vi "Read PortID.vi"(8 "error in (no error)":errorcluster, 11 "FlexLogger_gRPC in":refnum<class "FlexLogger_gRPC.lvclass">) -> (0 "error out":errorcluster, 2 "PortID":u32, 3 "FlexLogger_gRPC out":refnum<class "FlexLogger_gRPC.lvclass">)   [LabVIEW 2020, in "FlexLogger_gRPC.lvlib" / "FlexLogger_gRPC.lvclass"]
uses:
  FlexLogger_gRPC.lvclass
  FlexLogger_gRPC.lvclass/FlexLogger_gRPC.ctl
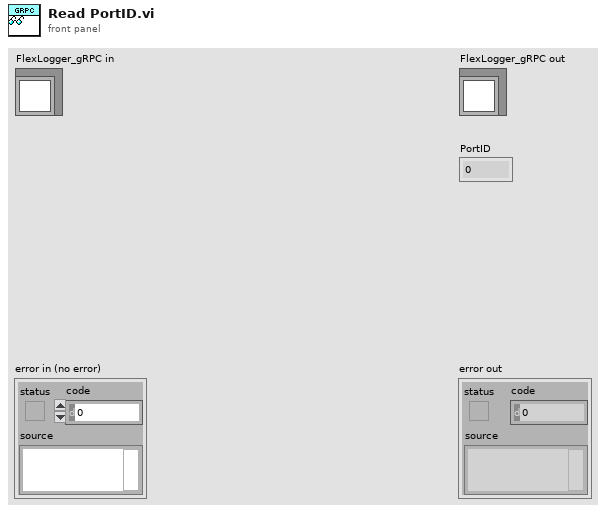
[diagram p1: front panel]
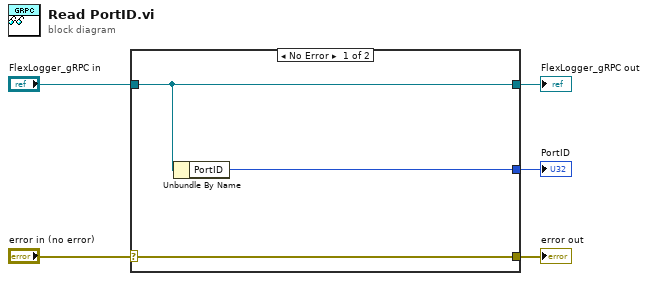
[diagram p0: block diagram]
diagram:
  n1 = case shown="No Error" "error in (no error)" {
    selector: "error in (no error)" -> [w8 w9]
    tunnel: [w8 w9] -> w4
    tunnel: [w7 w10] -> w2
    tunnel: "FlexLogger_gRPC in" -> [w7 w10]
    tunnel: [w6 _] -> w1
    frame No Error {
      n2 = Unbundle By Name(w7) -> ("PortID"=w6:u32)
    }
    frame Error {
    }
  }
  "error out" <- w4
  "FlexLogger_gRPC out" <- w2
  "PortID" <- w1
